vi "WriteDataToFile.vi"(8 "error in (no error)":errorcluster, 10 "Save Data":T1, 11 "File ref in":refnum<k34>) -> (0 "error out":errorcluster, 3 "File ref out":refnum<k34>)   [LabVIEW 2019]
uses:
  Typedefs/Saving Thread/#cluster_SaveData.ctl
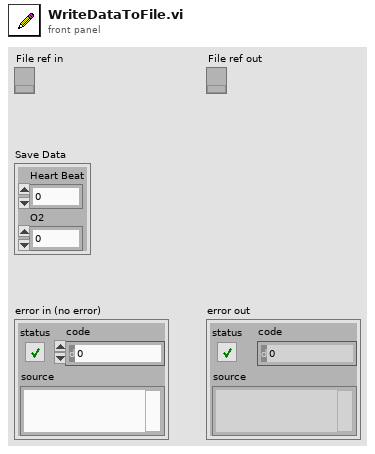
[diagram p1: front panel]
types:
  T1 = typedef "#cluster_SaveData.ctl" = cluster{"Heart Beat":dbl, "O2":dbl}
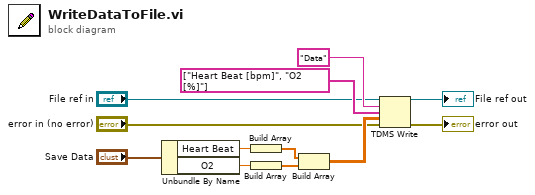
[diagram p0: block diagram]
diagram:
  n1 = Unbundle By Name("Save Data") -> ("Heart Beat"=w10:dbl, "O2"=w11:dbl)
  n2 = Build Array(w10) -> (w2:dbl[])
  n3 = Build Array(w11) -> (w1:dbl[])
  n4 = Build Array(w2, w1) -> (w12:dbl[][])
  n5 = TDMS Write(0:"File ref in", 5:"Data" ("group name in (Untitled)"), 7:string[] ["Heart Beat [bpm]", "O2 [%]"] ("channel name(s) in (Untitled)"), 9:w12, 11:"error in (no error)") -> (4:→"File ref out":refnum<k34>, 15:→"error out":errorcluster)  [unwired: 1 in, 2 out]
